vi "Mux8Way16.vi"(0 "c":bool[](array[boolean]), 1 "b":bool[](array[boolean]), 2 "a":bool[](array[boolean]), 5 "d":bool[](array[boolean]), 7 "e":bool[](array[boolean]), 9 "f":bool[](array[boolean]), 11 "g":bool[](array[boolean]), 12 "h":bool[](array[boolean]), 13 "sel":bool[](array[boolean])) -> (8 "out":bool[](array[boolean]))   [LabVIEW 2014]
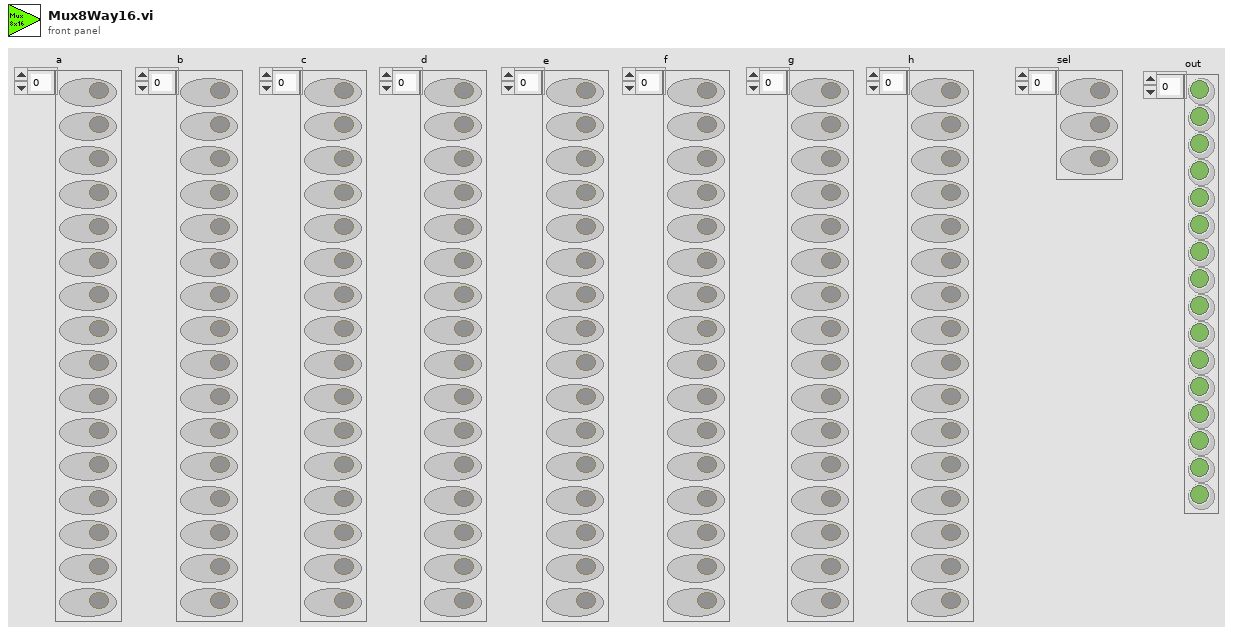
[diagram p1: front panel]
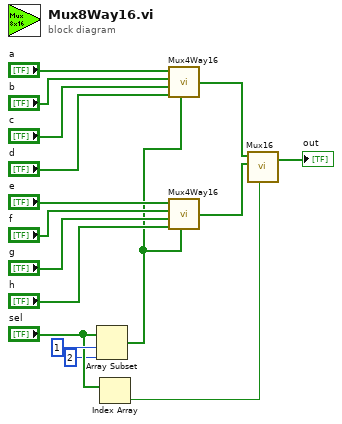
[diagram p0: block diagram]
diagram:
  n1 = Array Subset(array="sel", index=1, length=2) -> (w2:bool[])
  n2 = Index Array(array="sel") -> (element=w1:bool)  [unwired: 1 in]
  n3 = call "Mux4Way16.vi"("sel"=w2, "d"="d", "c"="c", "b"="b", "a"="a") -> ("out"=w5:bool[])  [unwired: 1 in]
  n4 = call "Mux4Way16.vi"("sel"=w2, "d"="h", "c"="g", "b"="f", "a"="e") -> ("out"=w4:bool[])  [unwired: 1 in]
  n5 = call "Mux16.vi"("sel"=w1, "b"=w4, "a"=w5) -> ("out"=→"out":bool[])  [unwired: 4 in]
